vi "login.vi"() -> ()   [LabVIEW 2021]
uses:
  <vilib>/Utility/file.llb/Write Delimited Spreadsheet (DBL).vi
panel:
  in  "?":enum32{"Login", "Personal Info"}(tab)
  out "Boolean":bool
  in  "Data":string[][](table)
  in  "Delete":bool
  in  "Add":bool
  in  "Login":bool
  in  "Password":string
  in  "Username":string
  in  "Reset":bool
  in  "Save":bool
  in  "IC Number":string
  in  "Age":string
  in  "Address":string
  in  "Name":string
  # "Login Page"
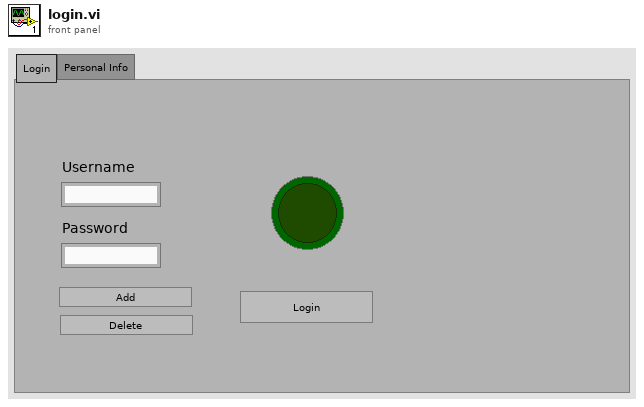
[diagram p1: front panel]
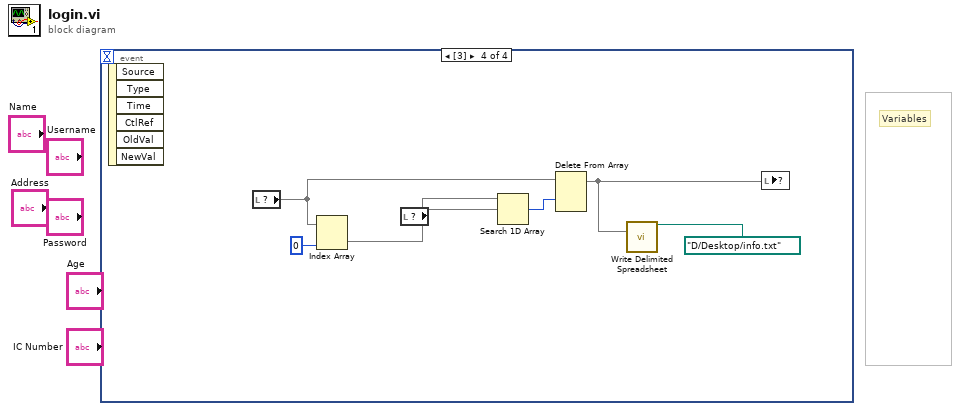
[diagram p0: block diagram]
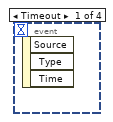
[diagram p2: hidden frame]
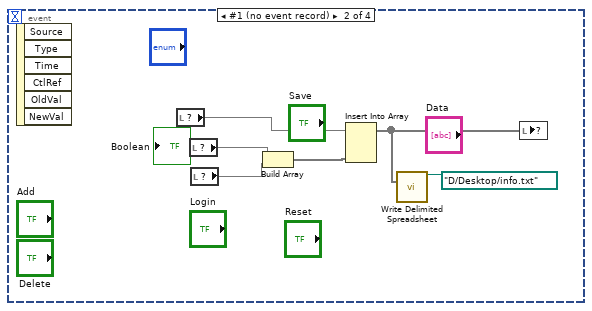
[diagram p3: hidden frame]
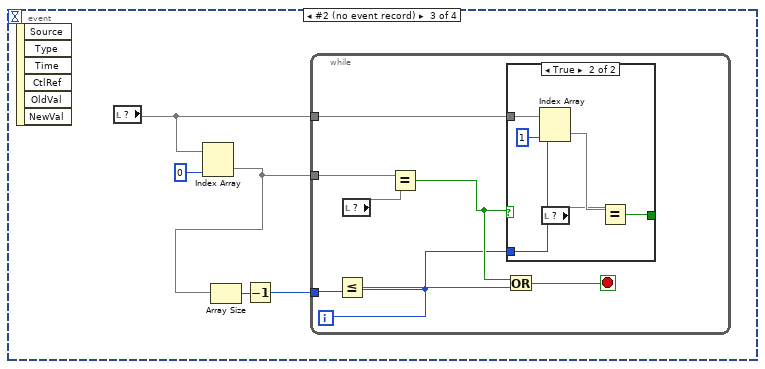
[diagram p4: hidden frame]
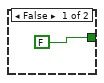
[diagram p5: hidden frame]
diagram:
  # "Variables"
  n1 = event shown="[3]" {
    selector: _ -> [_ _ _ _]
    dyn-events: _ -> [_ _ _ _]
    timeout: _ -> [_ _ _ _]
    event Timeout {
      n2 = event-data() -> ()  [unwired: 1 in, 3 out]
    }
    event #1 (no event record) {
      n3 = event-data() -> ()  [unwired: 1 in, 6 out]
      n4 = local read item#-1() -> (w6)
      n5 = local read item#-1() -> (w1)
      n6 = local read item#-1() -> (w2)
      n7 = Build Array(w1, w2) -> (w5:void[])
      n8 = Insert Into Array(array=w6, new element=w5) -> (w3:void[])  [unwired: 2 in]
      n9 = call-poly <vilib>:"Write Delimited Spreadsheet.vi"("file path (dialog if empty)"=path "D:/Desktop/info.txt", "2D data"=w3) -> ()  [unwired: 12 in, 2 out]
      n10 = local write item#-1(w3) -> ()
    }
    event #2 (no event record) {
      n11 = event-data() -> ()  [unwired: 1 in, 6 out]
      n12 = local read item#-1() -> (w7)
      n13 = Index Array "Index Array"(array=w7, index (col)=0) -> (element=w10)  [unwired: 1 in]
      n14 = Array Size(array=w10) -> (size(s)=w9:i32)
      n15 = Decrement(x=w9) -> (x-1=w8:i32)
      n16 = while {
        tunnel: w10 -> [w19]
        tunnel: w7 -> [w18]
        tunnel: w8 -> [w17]
        i -> [w12]
        stop <- w15 stop-if-true
        n17 = Less Or Equal?(x=w17, y=w12) -> (x <= y?=w13:bool)
        n18 = local read item#-1() -> (w14)
        n19 = Equal?(x=w19, y=w14) -> (x = y?=w16:bool)
        n20 = Or(x=w16, y=w13) -> (x .or. y?=w15:bool)
        n21 = case shown="True" w16 {
          tunnel: w18 -> [_ w26]
          tunnel: [FALSE w23] -> _
          tunnel: w12 -> [_ w22]
          frame False {
          }
          frame True {
            n22 = Index Array "Index Array"(array=w26, index (row)=w22, index (col)=1) -> (element=w24)
            n23 = local read item#-1() -> (w21)
            n24 = Equal?(x=w24, y=w21) -> (x = y?=w23:bool)
          }
        }
      }
    }
    event #3 (no event record) {
      n25 = event-data() -> ()  [unwired: 1 in, 6 out]
      n26 = local read item#-1() -> (w29)
      n27 = Index Array(array=w29, index (col)=0) -> (element=w32)  [unwired: 1 in]
      n28 = local read item#-1() -> (w31)
      n29 = Search 1D Array(1D array=w32, element=w31) -> (index of element=w30:i32)  [unwired: 1 in]
      n30 = Delete From Array "Delete From Array"(array=w29, index (row)=w30) -> (array with subset deleted=w27)  [unwired: 2 in, 1 out]
      n31 = call-poly <vilib>:"Write Delimited Spreadsheet.vi"("file path (dialog if empty)"=path "D:/Desktop/info.txt", "2D data"=w27) -> ()  [unwired: 12 in, 2 out]
      n32 = local write item#-1(w27) -> ()
    }
  }
